vi "Process.vi"(8 "error in":errorcluster, 11 "ZMQ":refnum<class "ZMQ_SMO.lvclass">) -> (0 "error out":errorcluster, 3 "ZMQ out":refnum<class "ZMQ_SMO.lvclass">)   [LabVIEW 2016, in "ZMQ_SMO.lvclass"]
doc: "---------------------------------------------------------------\nJKI State Machine Objects™\nhttp://jki.net/state-machine-objects/\nCopyright (C) 2005-2015, JKI <info@jki.net>\nALL RIGHTS RESERVED"
uses:
  ZMQ_SMO.lvclass
  C:/Program Files (x86)/National Instruments/LabVIEW 2016/vi.lib/JKI/JKI SMO/SMO/SMO.lvclass
  <vilib>/JKI/JKI SMO/SMO/Typedefs/Parent Call--Enum.ctl
  <vilib>/addons/zeromq/socket_type.ctl
  <vilib>/addons/zeromq/zmq_context.lvclass
  <vilib>/addons/zeromq/zmq_socket.lvclass
  ZMQ_SMO.lvclass/ZMQ_SMO.ctl
  <vilib>/addons/zeromq/socket_options.ctl
  <vilib>/addons/zeromq/poll_type.ctl
  <vilib>/addons/zeromq/zmq_poll_scalar.vi
  <vilib>/JKI/JKI SMO/SMO/SMO.lvclass
  <vilib>/addons/zeromq/zeromq.lvlib
panel:
  # "For instructions on how to use the JKI State Machine Objects, examples and video tutorials, visit:\nhttp://jki.net/state-machine-objects/\n\nJKI State Machine Objects™\nhttp://jki.net/state-machine-objects/\nCopyright (C) 2005-2015, JKI <info@jki.net>\nALL RIGHTS RESERVED"
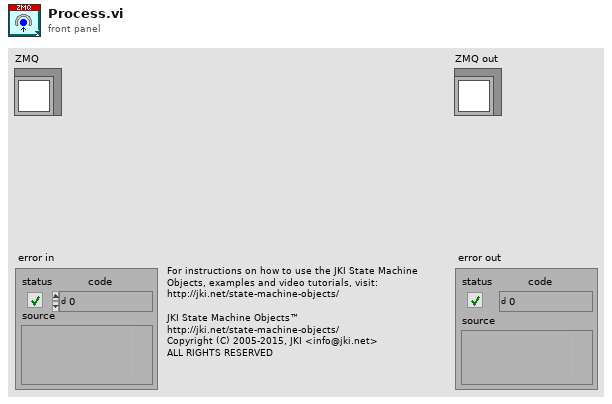
[diagram p1: front panel]
types:
  T1 = typedef "zeromq.lvlib/socket_type.ctl" = enum8{"ZMQ_PAIR", "ZMQ_PUB", "ZMQ_SUB", "ZMQ_REQ", "ZMQ_REP", "ZMQ_DEALER", "ZMQ_ROUTER", "ZMQ_PULL", "ZMQ_PUSH", "ZMQ_XPUB", "ZMQ_XSUB"}
  T2 = typedef "SMO.lvclass/Parent Call--Enum.ctl" = enum16{"Allows parent to run", "Does not request parent to run"}
  T3 = enum32{"invalid app kind", "Development System", "Run Time System", "Student Edition", "Embedded LabVIEW", "Evaluation", "Custom"}
  T4 = enum32{"Invalid", "Standard", "Closed", "Hidden", "Minimized", "Maximized"}
  T5 = enum32{"Bad", "Idle", "Run top level", "Running"}
  T6 = typedef "zeromq.lvlib/socket_options.ctl" = enum8{"NONE", "ZMQ_HWM", "<2>", "ZMQ_SWAP", "ZMQ_AFFINITY", "ZMQ_IDENTITY", "ZMQ_SUBSCRIBE", "ZMQ_UNSUBSCRIBE", "ZMQ_RATE", "ZMQ_RECOVERY_IVL", "ZMQ_MCAST_LOOP", "ZMQ_SNDBUF", "ZMQ_RCVBUF", "ZMQ_RCVMORE", "ZMQ_FD", "ZMQ_EVENTS", "ZMQ_TYPE", "ZMQ_LINGER", "ZMQ_RECONNECT_IVL", "ZMQ_BACKLOG", "ZMQ_RECOVERY_IVL_MSEC", "ZMQ_RECONNECT_IVL_MAX", "ZMQ_MAXMSGSIZE", "ZMQ_SNDHWM", "ZMQ_RCVHWM", "ZMQ_MULTICAST_HOPS", "<26>", "ZMQ_RCVTIMEO", "ZMQ_SNDTIMEO", "<29>", "<30>", "ZMQ_IPV4ONLY", "ZMQ_LAST_ENDPOINT", "ZMQ_ROUTER_MANDATORY", "ZMQ_TCP_KEEPALIVE", "ZMQ_TCP_KEEPALIVE_CNT", "ZMQ_TCP_KEEPALIVE_IDLE", "ZMQ_TCP_KEEPALIVE_INTVL", "ZMQ_TCP_ACCEPT_FILTER", "ZMQ_DELAY_ATTACH_ON_CONNECT", "ZMQ_XPUB_VERBOSE"}
  T7 = typedef "zeromq.lvlib/poll_type.ctl" = enum16{"None", "In", "Out", "In/Out"}
  T8 = typedef "ZMQ_SMO.lvclass/PrivateEvents--ZMQ.ZMQ_PublicMethod.ctl" = string[]
  T9 = typedef "ZMQ_ZMQ.lvclass/ZMQ Config.ctl" = cluster{"socket type":T1, "endpoint":string, "filter":string}
  T10 = cluster{"Core":cluster{"Current VI Reference":refnum<vi>, "Close Panel on Exit?":bool, "error":errorcluster}, "Self Reference":refnum<class "ZMQ_SMO.lvclass">, "parts":string[], "ZMQ context":refnum<class "zmq_context.lvclass">, "ZMQ socket":refnum<class "zmq_socket.lvclass">, "Config":T9, "to":i32}
  T11 = cluster{"Current VI Reference":refnum<vi>, "Close Panel on Exit?":bool, "error":errorcluster}
  T12 = typedef "SMO.lvclass/Protected Events.ctl" = cluster{"StopProcesses":refnum<user-event>, "AbortProcesses":refnum<user-event>, "Config Changed":refnum<user-event>, "Dependency":refnum<user-event>}
  T13 = typedef "ZMQ_SMO.lvclass/PrivateEvents--Cluster.ctl" = cluster{"ZMQ_message":refnum<user-event>}
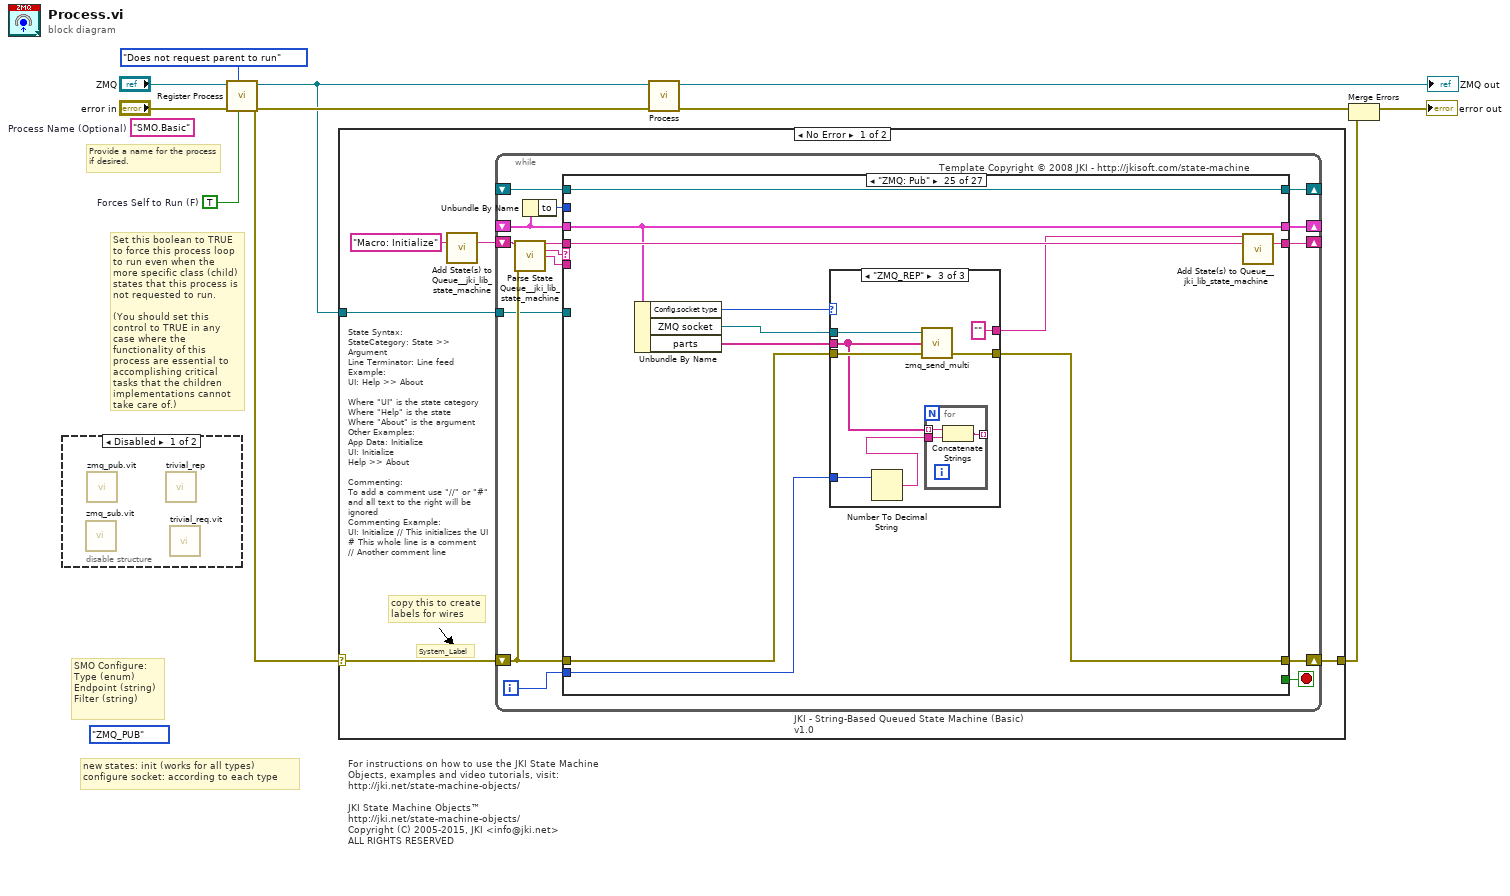
[diagram p0: block diagram]
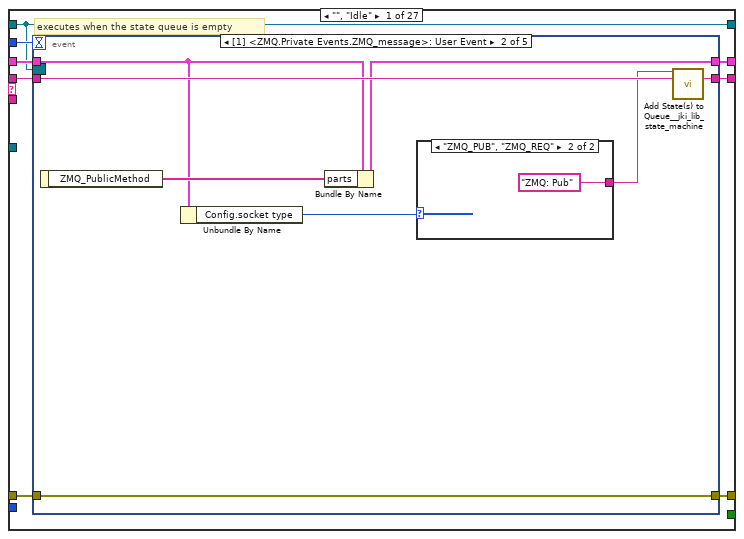
[diagram p3: hidden frame]
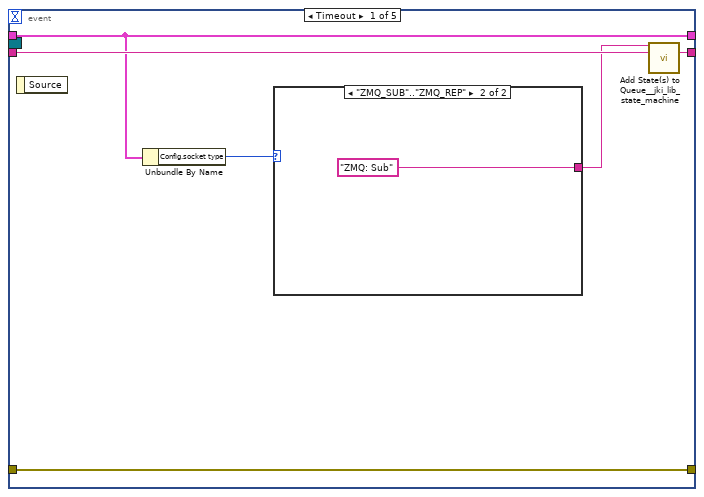
[diagram p4: hidden frame]
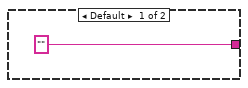
[diagram p5: hidden frame]
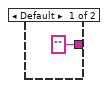
[diagram p6: hidden frame]
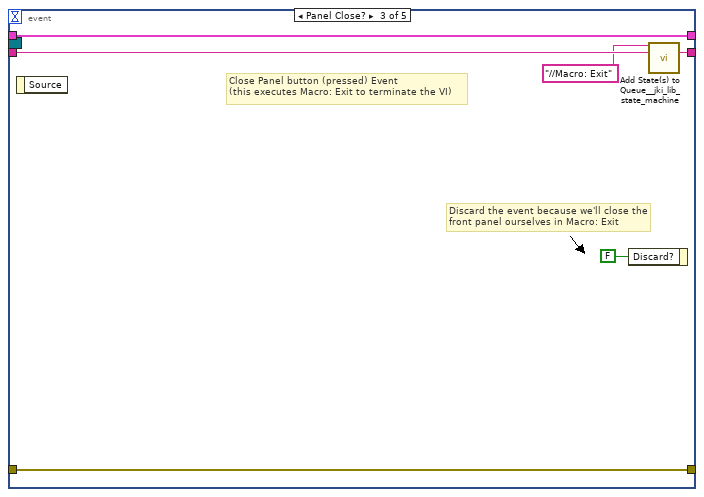
[diagram p7: hidden frame]
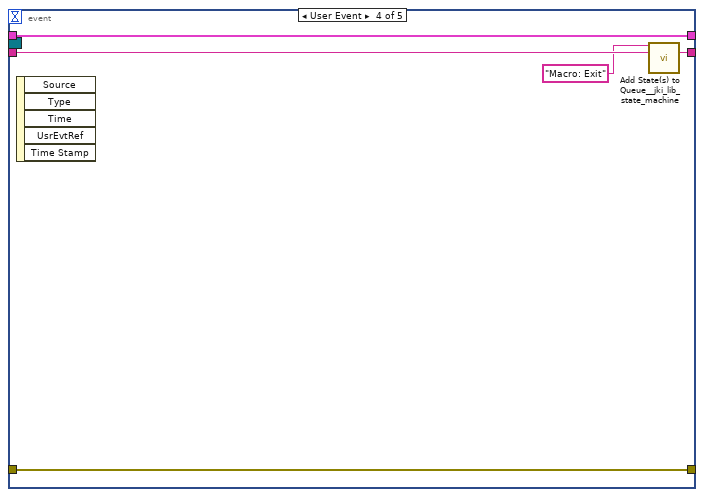
[diagram p8: hidden frame]
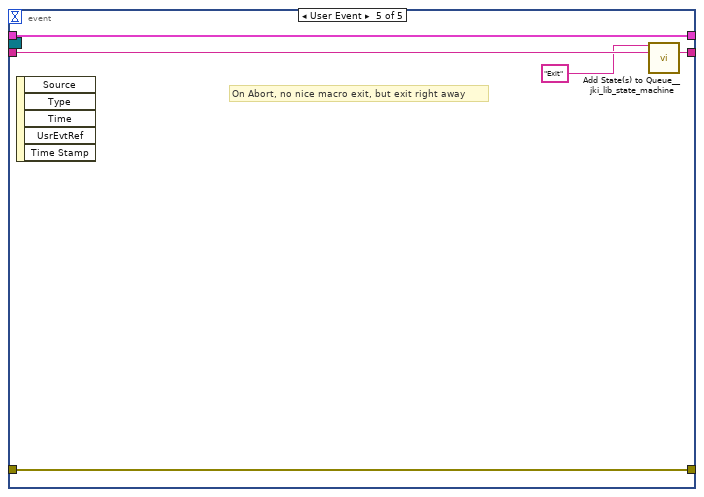
[diagram p9: hidden frame]
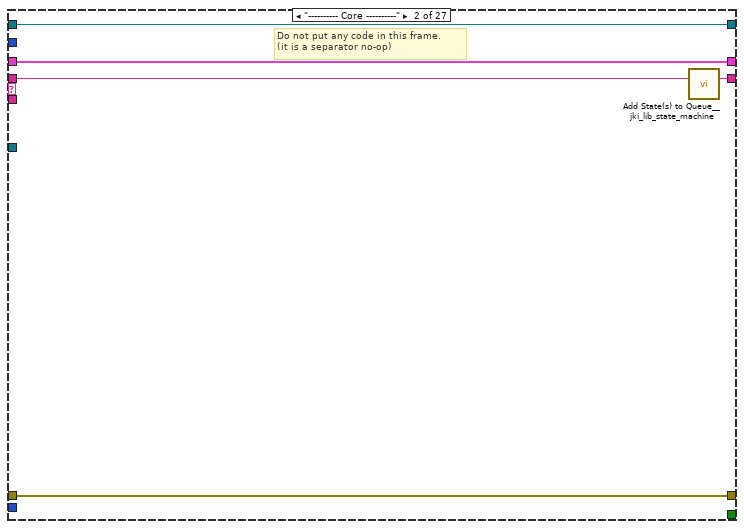
[diagram p10: hidden frame]
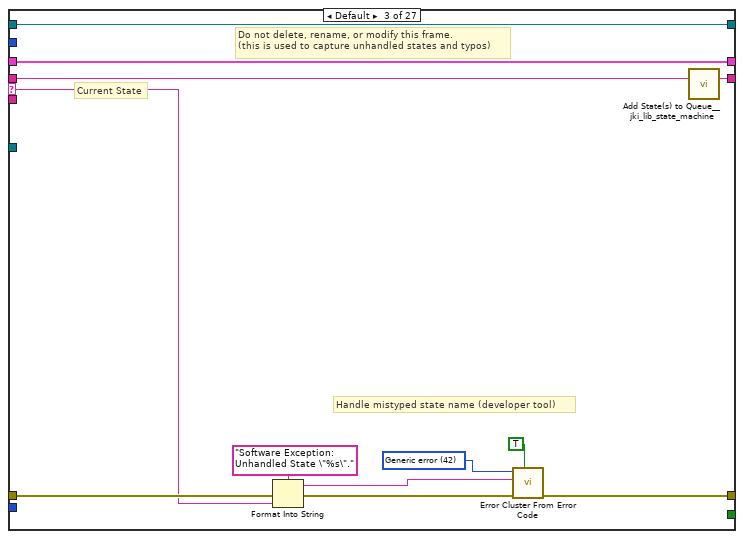
[diagram p11: hidden frame]
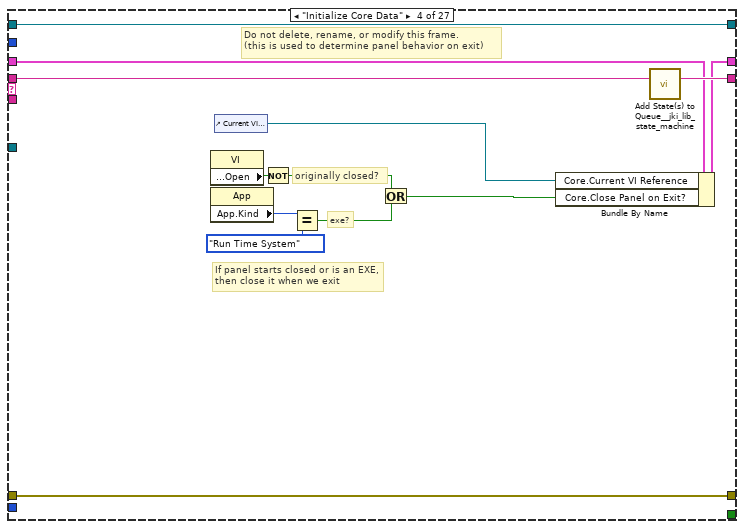
[diagram p12: hidden frame]
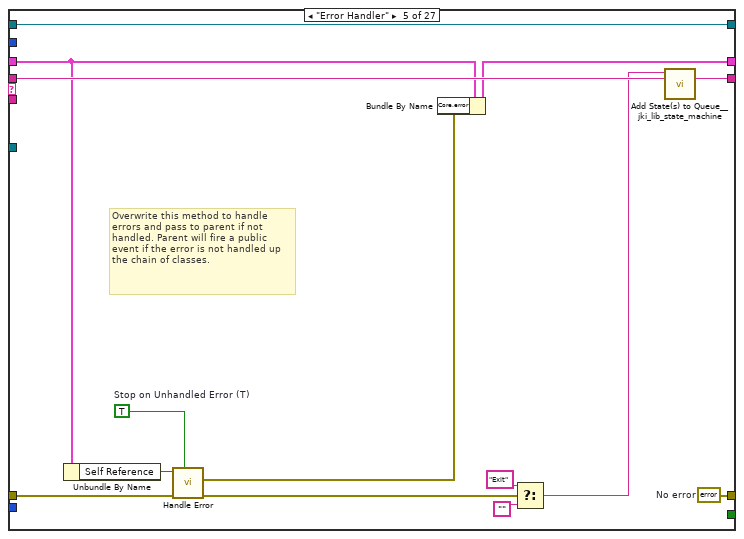
[diagram p13: hidden frame]
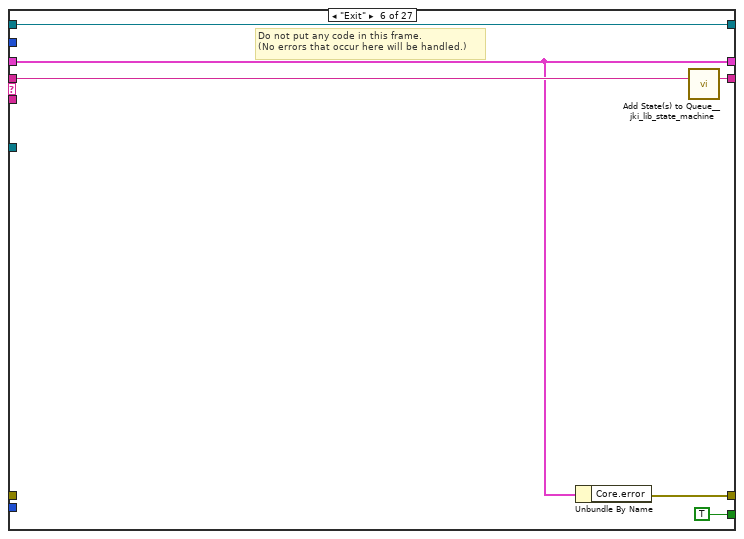
[diagram p14: hidden frame]
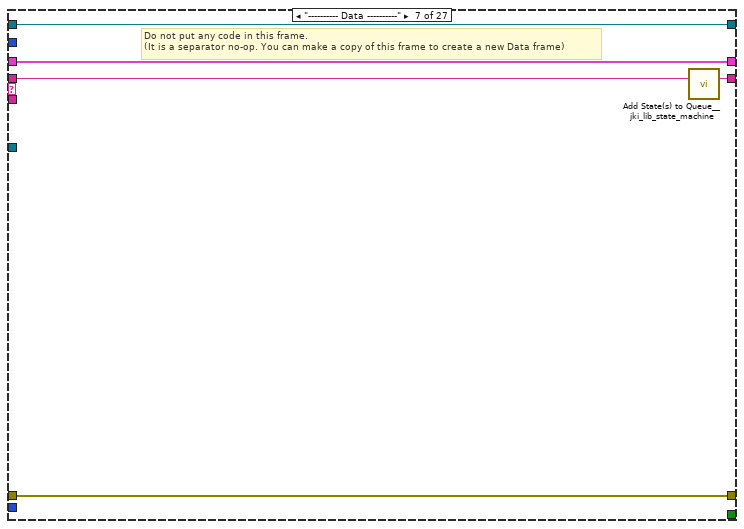
[diagram p15: hidden frame]
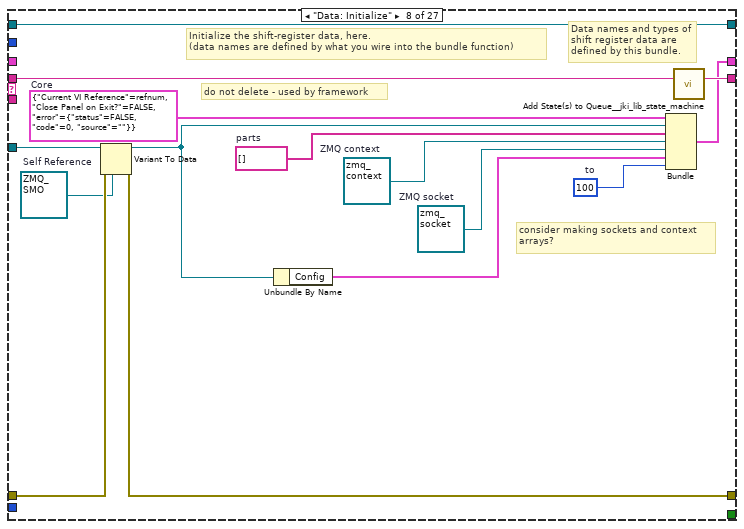
[diagram p16: hidden frame]
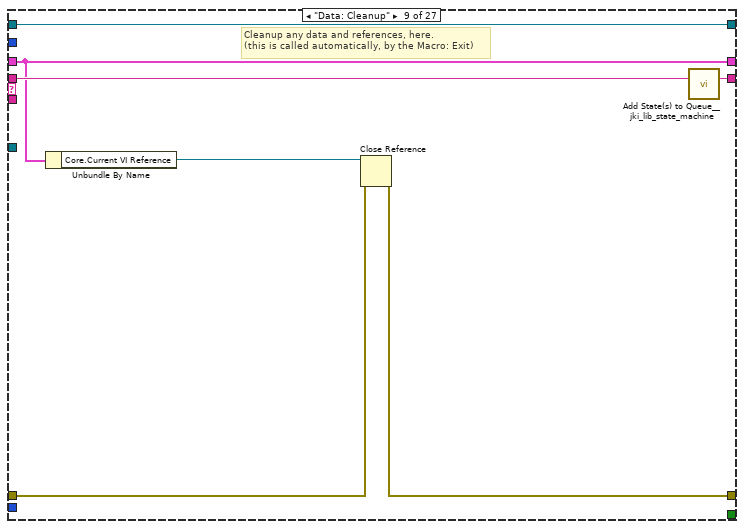
[diagram p17: hidden frame]
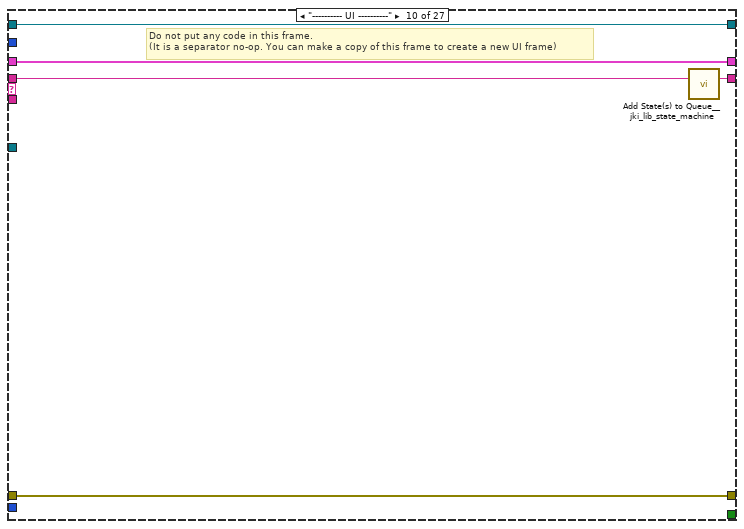
[diagram p18: hidden frame]
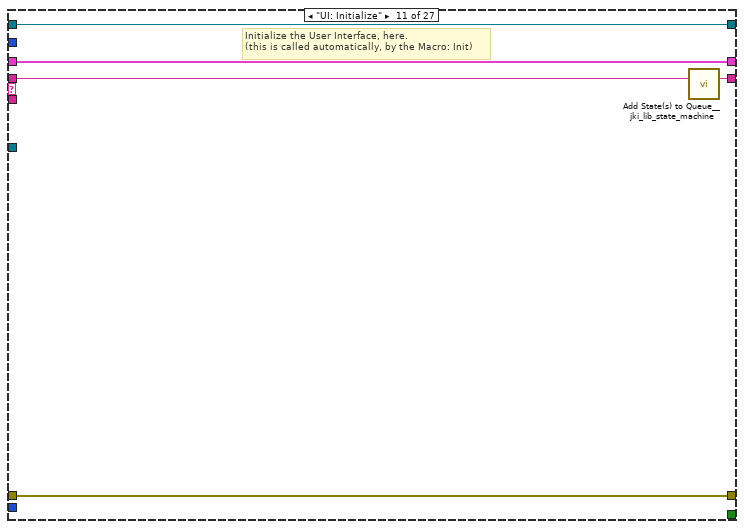
[diagram p19: hidden frame]
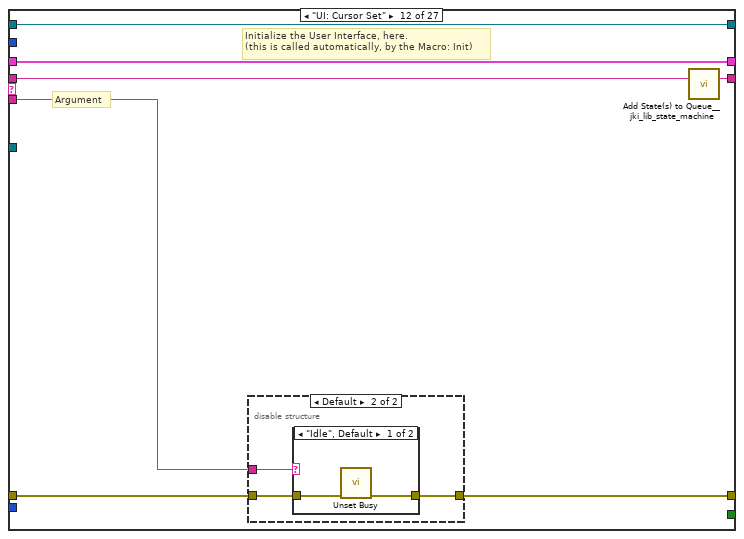
[diagram p20: hidden frame]
diagram:
  (unwired) socket_type."ZMQ_PUB" ("socket type")
  w1 = TRUE  # Forces Self to Run (F)
  (unwired) "SMO.Basic"  # Process Name (Optional)
  # "new states: init (works for all types)\nconfigure socket: according to each type"
  # "SMO Configure:\nType (enum)\nEndpoint (string)\nFilter (string)"
  # "Provide a name for the process\nif desired."
  # "Set this boolean to TRUE to force this process loop to run even when the more specific class (child) states that this process is not requested to run.\n\n(You should set this control to TRUE in any case where the functionality of this process are essential to accomplishing critical tasks that the children implementations cannot take care of.)"
  # "For instructions on how to use the JKI State Machine Objects, examples and video tutorials, visit:\nhttp://jki.net/state-machine-objects/\n\nJKI State Machine Objects™\nhttp://jki.net/state-machine-objects/\nCopyright (C) 2005-2015, JKI <info@jki.net>\nALL RIGHTS RESERVED"
  n1 = disable-structure shown="Disabled" {
    frame Disabled {
      n2 = call "zmq_sub.vit"() -> ()  [unwired: 12 in]
      n3 = call "zmq_pub.vit"() -> ()  [unwired: 12 in]
      n4 = call "trivial_rep.vi"() -> ()  [unwired: 12 in]
      n5 = call "trivial_req.vit"() -> ()  [unwired: 12 in]
    }
    frame Enabled {
    }
  }
  n6 = call <vilib>:"Register Process.vi"("Forces Self to Run (F)"=w1, "Parent Call"=Parent_Call--Enum."Does not request parent to run", "error in (no error)"="error in", "SMO"="ZMQ") -> ("error out"=w7:errorcluster, "SMO out"=w6:refnum<class "ZMQ_SMO.lvclass">)  [unwired: 6 in]
  n7 = case shown="No Error" w7 {
    selector: w7 -> [w12 w411]
    tunnel: w6 -> [w13 _]
    tunnel: [w11 w411] -> w3
    frame No Error {
      # "State Syntax:\nStateCategory: State >> Argument\nLine Terminator: Line feed\nExample:\nUI: Help >> About\n\nWhere \"UI\" is the state category\nWhere \"Help\" is the state\nWhere \"About\" is the argument\nOther Examples:\nApp Data: Initialize\nUI: Initialize\nHelp >> About\n\nCommenting:\nTo add a comment use \"//\" or \"#\" and all text to the right will be ignored\nCommenting Example:\nUI: Initialize // This initializes the UI\n# This whole line is a comment\n// Another comment line"
      # "copy this to create labels for wires"
      # "System_Label"
      n8 = call <vilib>:"Add State(s) to Queue__jki_lib_state_machine.vi"("State(s) in (\"\")"="Macro: Initialize") -> ("States Out"=w15:string)  [unwired: 14 in]
      n9 = while "JKI - String-Based Queued State Machine (Basic) v1.0" {
        shift-right: [w23] -> _
        shift-left: _ -> [w17]
        shift-right: [w26] -> w11
        shift-left: w12 -> [w22]
        shift-right: [w25] -> _
        shift-left: w15 -> [w27]
        tunnel: w13 -> [w21]
        shift-right: [w20] -> _
        shift-left: _ -> [w19]
        i -> [w16]
        stop <- w24 stop-if-true
        # "Template Copyright © 2008 JKI - http://jkisoft.com/state-machine"
        n10 = call <vilib>:"Parse State Queue__jki_lib_state_machine.vi"("State Queue"=w27, "Error In (no error)"=w22) -> ("Remaining States"=w29:string, "Current State"=w30:string, "Arguments"=w28:string)  [unwired: 11 in]
        n11 = Unbundle By Name(w17) -> ("to"=w18:i32)
        n12 = case shown="\"ZMQ: Pub\"" w30 {
          selector: w30 -> [_ _ w79 _ _ _ _ _ _ _ _ _ _ _ _ _ _ _ _ _ _ _ _ _ _ _ _]
          tunnel: w29 -> [w38 w77 w83 w102 w116 w122 w127 w142 w149 w154 w159 w166 w182 w214 w228 w242 w247 w258 w263 w276 w282 w287 w299 w312 w351 w381 w410]
          tunnel: w28 -> [_ _ _ _ _ _ _ _ _ _ _ w160 w176 _ _ _ _ _ _ _ _ _ _ _ _ _ _]
          tunnel: w17 -> [w36 w74 w81 w93 w110 w118 w124 _ w144 w151 w157 w164 w178 w211 w216 w233 w244 w255 w260 w274 w280 w285 w288 w308 w344 w378 w402]
          tunnel: [w35 w75 w85 w99 w111 w117 w125 w139 w145 w152 w156 w161 w179 w212 w226 w240 w245 w249 w261 w269 w278 w283 w292 w305 w345 w377 w405] -> w26
          tunnel: w22 -> [w34 w75 w84 w99 w112 _ w125 w140 w146 w152 w156 w162 w180 w212 w226 w240 w245 w250 w261 w270 w278 w283 w290 w306 w346 w371 w406]
          tunnel: [w37 w76 w82 w101 w115 w121 w126 w141 w148 w153 w158 w165 w181 w213 w227 w241 w246 w257 w262 w275 w281 w286 w298 w311 w350 w380 w409] -> w25
          tunnel: [_ _ _ _ _ TRUE _ _ _ _ _ _ _ _ _ _ _ _ _ _ _ _ _ _ _ _ _] -> w24
          tunnel: [w33 w74 w81 w100 w109 w118 w124 w128 w144 w151 w157 w164 w178 w211 w216 w233 w244 w255 w260 w274 w280 w285 w296 w309 w344 w378 w402] -> w23
          tunnel: w18 -> [w32 _ _ _ _ _ _ _ _ _ _ _ _ _ _ _ _ _ _ _ _ _ _ _ _ _ _]
          tunnel: w21 -> [_ _ _ _ _ _ _ w137 _ _ _ _ _ _ _ _ _ _ _ _ _ _ _ _ _ _ _]
          tunnel: [w31 w73 w78 w90 w114 w119 w123 w136 w143 w150 w155 w163 w175 w210 w225 w234 w243 w256 w259 w273 w279 w284 w297 w310 w349 w379 w408] -> w20
          tunnel: w19 -> [w31 w73 w78 w90 w114 w119 w123 w136 w143 w150 w155 w163 w175 w210 w225 w234 w243 w256 w259 _ w279 w284 w297 w310 w349 w379 w408]
          tunnel: w16 -> [_ _ _ _ _ _ _ _ _ _ _ _ _ _ _ _ _ _ _ _ _ _ _ _ w341 _ _]
          frame "", "Idle" {
            # "executes when the state queue is empty"
            n13 = event shown="[1] <ZMQ.Private Events.ZMQ_message>: User Event" {
              selector: w31 -> [_ _ _ _ _]
              dyn-events: _ -> [_ _ _ _ _]
              timeout: w32 -> [_ _ _ _ _]
              tunnel: w38 -> [w44 w54 w62 w67 w72]
              tunnel: [w43 w53 w61 w66 w71] -> w37
              tunnel: w36 -> [w42 w48 w59 w64 w69]
              tunnel: [w40 w49 w60 w65 w70] -> w35
              tunnel: w34 -> [w40 w49 w60 w65 w70]
              tunnel: [w42 w52 w59 w64 w69] -> w33
              event Timeout {
                n14 = event-data() -> ()  [unwired: 1 in, 1 out]
                n15 = Unbundle By Name(w42) -> ("Config.socket type"=w41:T1)
                n16 = case shown="\"ZMQ_SUB\"..\"ZMQ_REP\"" w41 {
                  tunnel: ["" ("string") "ZMQ: Sub" ("string")] -> w39
                  frame Default {
                  }
                  frame "ZMQ_SUB".."ZMQ_REP" {
                  }
                }
                n17 = call <vilib>:"Add State(s) to Queue__jki_lib_state_machine.vi"("State(s) in Front (\"\")"=w39, "State(s) in (\"\")"=w44) -> ("States Out"=w43:string)  [unwired: 13 in]
              }
              event User Event {
                n18 = event-data() -> ("ZMQ_PublicMethod"=w51:T8)  [unwired: 1 in]
                n19 = Unbundle By Name(w48) -> ("Config.socket type"=w47:T1)
                n20 = Bundle By Name(cluster=w48, "parts"=w51) -> (w52:T10)
                n21 = case shown="\"ZMQ_PUB\", \"ZMQ_REQ\"" w47 {
                  tunnel: ["" ("string") "ZMQ: Pub" ("string")] -> w50
                  frame Default {
                  }
                  frame "ZMQ_PUB", "ZMQ_REQ" {
                  }
                }
                n22 = call <vilib>:"Add State(s) to Queue__jki_lib_state_machine.vi"("State(s) in Front (\"\")"=w50, "State(s) in (\"\")"=w54) -> ("States Out"=w53:string)  [unwired: 13 in]
              }
              event Panel Close? {
                # "Discard the event because we'll close the front panel ourselves in Macro: Exit"
                # "Close Panel button (pressed) Event\n(this executes Macro: Exit to terminate the VI)"
                n23 = event-data() -> ()  [unwired: 1 in, 1 out]
                n24 = event-data("Discard?"=FALSE) -> ()  [unwired: 1 in, 1 out]
                n25 = call <vilib>:"Add State(s) to Queue__jki_lib_state_machine.vi"("State(s) in Front (\"\")"="//Macro: Exit", "State(s) in (\"\")"=w62) -> ("States Out"=w61:string)  [unwired: 13 in]
              }
              event User Event {
                n26 = event-data() -> ()  [unwired: 1 in, 5 out]
                n27 = call <vilib>:"Add State(s) to Queue__jki_lib_state_machine.vi"("State(s) in Front (\"\")"="Macro: Exit", "State(s) in (\"\")"=w67) -> ("States Out"=w66:string)  [unwired: 13 in]
              }
              event User Event {
                # "On Abort, no nice macro exit, but exit right away"
                n28 = event-data() -> ()  [unwired: 1 in, 5 out]
                n29 = call <vilib>:"Add State(s) to Queue__jki_lib_state_machine.vi"("State(s) in Front (\"\")"="Exit", "State(s) in (\"\")"=w72) -> ("States Out"=w71:string)  [unwired: 13 in]
              }
            }
          }
          frame "---------- Core ----------" {
            # "Do not put any code in this frame.\n(it is a separator no-op)"
            n30 = call <vilib>:"Add State(s) to Queue__jki_lib_state_machine.vi"("State(s) in (\"\")"=w77) -> ("States Out"=w76:string)  [unwired: 14 in]
          }
          frame Default {
            w88 = 42 items=["No error", "Argument error", "Memory is full", "Out of zone", "End of file", "File already open", "Generic file I/O error", "File not found", "File permission error", "Disk is full", "Duplicate path", "Too many files open", "System feature not enabled", "Resource file not found", "Cannot add resource", "Resource not found", "Image not found", "Image memory error", "Pen does not exist", "Config type invalid", "Config token not found", "Config parse error", "Config memory error", "Bad external code format", "Bad external code offset", "External code not present", "Null window", "Destroy window error", "Null menu", "Print aborted", "Bad print record", "Print driver error", "Windows error during printing", "Memory error during printing", "Print dialog error", "Generic print error", "Invalid device refnum", "Device not found", "Device parameter error", "Device unit error", "Cannot open device", "Device call aborted", "Generic error", "Cancelled by user", "Object ID too low", "Object ID too high", "Object not in heap", "Unknown heap", "Unknown object (invalid DefProc)", "Unknown object (DefProc not in table)", "Message out of range", "Invalid (null) method", "Unknown message", "Manager call not supported", "Bad address", "Network operation in progress", "Network operation timed out", "Connection is busy", "Network attribute not supported", "Network error", "Address in use", "System out of memory", "Connection aborted", "Connection refused", "Not connected", "Already connected", "Connection closed", "Initialization error (interapplication manager)", "Bad occurrence", "Wait on unbound occurrence handler", "Occurrence queue overflow", "Datalog type conflict", "Unused", "Unrecognized type (interapplication manager)", "Memory corrupt", "Failed to make temporary DLL", "Old CIN version", "Drag socket not found", "Failed to load drop-object", "Failed to register OLE object", "Failed to release OLE object", "Format specifier type mismatch", "Unknown format specifier", "Too few format specifiers", "Too many format specifiers", "Scan failed", "Newer CIN version", "Error converting to variant", "Runtime menu error", "Password tampered", "Variant attribute not found", "Incompatible variant data type", "Event data is not available", "Event Store is not present", "Occurrence is not found", "Event Queue is not created", "Event info is not available", "Refnum passed is NULL", "Error retrieving Class GUID", "Error retrieving CoClass GUID", "Error retrieving TypeLib GUID.", "Bad built application magic bytes.", "Specific driver is different from the specific driver associated with the Logical Name.", "There is no session opened to the class driver.", "Max Error", "MAX - Error with config objects", "MAX - Error loading configuration", "MAX - Group not supported"]
            # "Current State"
            # "Do not delete, rename, or modify this frame.\n(this is used to capture unhandled states and typos)"
            # "Handle mistyped state name (developer tool)"
            n31 = Format Into String(format string="Software Exception: Unhandled State \"%s\"." ("message"), error in=w84, w79) -> (resulting string=w87:string, error out=w86:errorcluster)  [unwired: 1 in]
            n32 = call <vilib>:"Error Cluster From Error Code.vi"("show call chain? (False)"=TRUE, "error in (no error)"=w86, "error message (\"\")"=w87, "error code (0)"=w88) -> ("error out"=w85:errorcluster)  [unwired: 5 in]
            n33 = call <vilib>:"Add State(s) to Queue__jki_lib_state_machine.vi"("State(s) in (\"\")"=w83) -> ("States Out"=w82:string)  [unwired: 14 in]
          }
          frame "Initialize Core Data" {
            # "Do not delete, rename, or modify this frame.\n(this is used to determine panel behavior on exit)"
            # "originally closed?"
            # "exe?"
            # "If panel starts closed or is an EXE, then close it when we exit"
            n34 = property class="VI"() -> ("Front Panel.Open"=w98:bool)  [unwired: 2 in, 2 out]
            n35 = property class="App"() -> ("App.Kind"=w97:T3)  [unwired: 2 in, 2 out]
            n36 = control-ref of="Current VI Reference"() -> (w91:refnum<vi>)
            n37 = Not(x=w98) -> (.not. x?=w95:bool)
            n38 = Equal?(x=w97, y=T3."Run Time System" ("Application:Kind")) -> (x = y?=w94:bool)
            n39 = Or(x=w95, y=w94) -> (x .or. y?=w92:bool)
            n40 = Bundle By Name(cluster=w93, "Core.Current VI Reference"=w91, "Core.Close Panel on Exit?"=w92) -> (w100:T10)
            n41 = call <vilib>:"Add State(s) to Queue__jki_lib_state_machine.vi"("State(s) in (\"\")"=w102) -> ("States Out"=w101:string)  [unwired: 14 in]
          }
          frame "Error Handler" {
            w103 = TRUE  # Stop on Unhandled Error (T)
            w111 = errorcluster {"status"=FALSE, "code"=0, "source"=""}  # No error
            # "Overwrite this method to handle errors and pass to parent if not handled. Parent will fire a public event if the error is not handled up the chain of classes."
            n42 = Unbundle By Name(w110) -> ("Self Reference"=w113:refnum<class "ZMQ_SMO.lvclass">)
            n43 = call-dynamic "Handle Error.vi"("Stop on Unhandled Error (T)"=w103, "error in"=w112, "SMO"=w113) -> ("handling error"=w104:errorcluster, "Unhandled error"=w107:errorcluster)  [unwired: 6 in, 1 out]
            n44 = Bundle By Name(cluster=w110, "Core.error"=w107) -> (w109:T10)
            n45 = Select(t="Exit", s=w104, f="") -> (s? t:f=w108:string)
            n46 = call <vilib>:"Add State(s) to Queue__jki_lib_state_machine.vi"("State(s) in Front (\"\")"=w108, "State(s) in (\"\")"=w116) -> ("States Out"=w115:string)  [unwired: 13 in]
          }
          frame "Exit" {
            # "Do not put any code in this frame.\n(No errors that occur here will be handled.)"
            n47 = Unbundle By Name(w118) -> ("Core.error"=w117:errorcluster)
            n48 = call <vilib>:"Add State(s) to Queue__jki_lib_state_machine.vi"("State(s) in (\"\")"=w122) -> ("States Out"=w121:string)  [unwired: 14 in]
          }
          frame "---------- Data ----------" {
            # "Do not put any code in this frame.\n(It is a separator no-op. You can make a copy of this frame to create a new Data frame)"
            n49 = call <vilib>:"Add State(s) to Queue__jki_lib_state_machine.vi"("State(s) in (\"\")"=w127) -> ("States Out"=w126:string)  [unwired: 14 in]
          }
          frame "Data: Initialize" {
            w129 = 100  # to
            w130 = string[] []  # parts
            w133 = refnum<class "zmq_socket.lvclass"> refnum  # ZMQ socket
            w134 = refnum<class "zmq_context.lvclass"> refnum  # ZMQ context
            w135 = T11 {"Current VI Reference"=refnum, "Close Panel on Exit?"=FALSE, "error"={"status"=FALSE, "code"=0, "source"=""}}  # Core
            w138 = refnum<class "ZMQ_SMO.lvclass"> refnum  # Self Reference
            # "consider making sockets and context\narrays?"
            # "do not delete - used by framework"
            # "Data names and types of shift register data are defined by this bundle."
            # "Initialize the shift-register data, here.\n(data names are defined by what you wire into the bundle function)"
            n50 = Variant To Data(error in=w140, type=w138, Variant=w137) -> (data=w132:refnum<class "ZMQ_SMO.lvclass">, error out=w139:errorcluster)
            n51 = Unbundle By Name(w132) -> ("Config"=w131:T9)
            n52 = Bundle("Core"=w135, "Self Reference"=w132, "parts"=w130, "ZMQ context"=w134, "ZMQ socket"=w133, "Config"=w131, "to"=w129) -> (w128:T10)  [unwired: 1 in]
            n53 = call <vilib>:"Add State(s) to Queue__jki_lib_state_machine.vi"("State(s) in (\"\")"=w142) -> ("States Out"=w141:string)  [unwired: 14 in]
          }
          frame "Data: Cleanup" {
            # "Cleanup any data and references, here.\n(this is called automatically, by the Macro: Exit)"
            n54 = Unbundle By Name(w144) -> ("Core.Current VI Reference"=w147:refnum<vi>)
            n55 = Close Reference(reference=w147, error in (no error)=w146) -> (error out=w145:errorcluster)
            n56 = call <vilib>:"Add State(s) to Queue__jki_lib_state_machine.vi"("State(s) in (\"\")"=w149) -> ("States Out"=w148:string)  [unwired: 14 in]
          }
          frame "---------- UI ----------" {
            # "Do not put any code in this frame.\n(It is a separator no-op. You can make a copy of this frame to create a new UI frame)"
            n57 = call <vilib>:"Add State(s) to Queue__jki_lib_state_machine.vi"("State(s) in (\"\")"=w154) -> ("States Out"=w153:string)  [unwired: 14 in]
          }
          frame "UI: Initialize" {
            # "Initialize the User Interface, here.\n(this is called automatically, by the Macro: Init)"
            n58 = call <vilib>:"Add State(s) to Queue__jki_lib_state_machine.vi"("State(s) in (\"\")"=w159) -> ("States Out"=w158:string)  [unwired: 14 in]
          }
          frame "UI: Cursor Set" {
            # "Argument"
            # "Initialize the User Interface, here.\n(this is called automatically, by the Macro: Init)"
            n59 = disable-structure shown="Default" {
              disable-tunnel: w162 -> [w167 w170]
              disable-tunnel: [w167 w169] -> w161
              disable-tunnel: w160 -> [_ w168]
              frame condition #0 {
              }
              frame condition #1 (active) {
                n60 = case shown="\"Idle\", Default" w168 {
                  tunnel: w170 -> [w172 w174]
                  tunnel: [w171 w173] -> w169
                  frame "Idle", Default {
                    n61 = call <vilib>:"Unset Busy.vi"("error in (no error)"=w172) -> ("error out"=w171:errorcluster)  [unwired: 10 in]
                  }
                  frame "Busy" {
                    n62 = call <vilib>:"Set Busy.vi"("error in (no error)"=w174) -> ("error out"=w173:errorcluster)  [unwired: 9 in, 1 out]
                  }
                }
              }
            }
            n63 = call <vilib>:"Add State(s) to Queue__jki_lib_state_machine.vi"("State(s) in (\"\")"=w166) -> ("States Out"=w165:string)  [unwired: 14 in]
          }
          frame "UI: Front Panel State" {
            # "Argument"
            # "Set Front Panel Open or Closed\n(Usage: \"UI: Front Panel State >> Open|Close\")"
            n64 = Unbundle By Name(w178) -> ("Core.Current VI Reference"=w177:refnum<vi>)
            n65 = disable-structure shown="Default" {
              disable-tunnel: w180 -> [w186 w209]
              disable-tunnel: [w185 w209] -> w179
              disable-tunnel: w177 -> [w184 _]
              disable-tunnel: w176 -> [w183 _]
              frame condition #0 (active) {
                n66 = case shown="\"Close\"" w183 {
                  tunnel: w186 -> [w190 w203]
                  tunnel: [w192 w204] -> w185
                  tunnel: w184 -> [w191 w201]
                  frame "Open", Default {
                    n67 = property class="VI"(reference=w191, error in=w190) -> (reference out=w188:refnum<vi>, error out=w189:errorcluster, "FP.State"=w187:T4)
                    n68 = case shown="\"Closed\"" w187 {
                      tunnel: [w195 w198] -> w192
                      tunnel: w189 -> [w194 w198]
                      tunnel: w188 -> [w193 _]
                      frame "Closed" {
                        n69 = invoke class="VI" method="FP.Open"(reference=w193, error in=w194, "Activate"=TRUE, "State"=T4."Standard") -> (error out=w195:errorcluster)  [unwired: 1 in, 4 out]
                      }
                      frame Default {
                      }
                    }
                  }
                  frame "Close" {
                    n70 = property class="VI"(reference=w201, error in=w203) -> (reference out=w200:refnum<vi>, error out=w202:errorcluster, "FP.State"=w199:T4)
                    n71 = case shown="Default" w199 {
                      tunnel: [w205 w208] -> w204
                      tunnel: w202 -> [w205 w207]
                      tunnel: w200 -> [_ w206]
                      frame "Invalid", "Closed" {
                      }
                      frame Default {
                        n72 = invoke class="VI" method="FP.Close"(reference=w206, error in=w207) -> (error out=w208:errorcluster)  [unwired: 1 in, 2 out]
                      }
                    }
                  }
                }
              }
              frame condition #1 {
              }
            }
            n73 = call <vilib>:"Add State(s) to Queue__jki_lib_state_machine.vi"("State(s) in (\"\")"=w182) -> ("States Out"=w181:string)  [unwired: 14 in]
          }
          frame "---------- Macro ----------" {
            # "Do not put any code in this frame.\n(It is a separator no-op. You can make a copy of this frame to create a new Macro frame)"
            n74 = call <vilib>:"Add State(s) to Queue__jki_lib_state_machine.vi"("State(s) in (\"\")"=w214) -> ("States Out"=w213:string)  [unwired: 14 in]
          }
          frame "Macro: Initialize" {
            w221 = "UI: Initialize\nUI: Front Panel State >> Close\nZMQ: Init\nZMQ: Config"  # UI: Initialize UI: Front Panel State >> Close ZMQ: Init ZMQ: Config
            w217 = "Process: Sync"
            # "Initialization Macro\n(This is called once, when the VI starts)"
            n75 = control-ref of="This VI"() -> (w219:refnum<vi>)
            n76 = property class="VI"(reference=w219) -> ("Exec.State"=w218:T5)  [unwired: 1 in, 2 out]
            n77 = Equal?(x=w218, y=T5."Run top level") -> (x = y?=w223:bool)
            n78 = Select(t=w217, s=w223, f="") -> ()  [unwired: 1 out]
            n79 = call <vilib>:"Add State(s) to Queue__jki_lib_state_machine.vi"("State(s) in Front (\"\")"="Data: Initialize\nInitialize Core Data\nEvents: Register", "State(s) in (\"\")"=w217, "State(s) at Back (\"\")"=w221) -> ("States Out"=w220:string)  [unwired: 12 in]
            n80 = call <vilib>:"Add State(s) to Queue__jki_lib_state_machine.vi"("State(s) in Front (\"\")"=w220, "State(s) in (\"\")"=w228) -> ("States Out"=w227:string)  [unwired: 13 in]
          }
          frame "Macro: Exit" {
            # "Exit Macro\n(This is called once, when the VI exits)"
            n81 = Unbundle By Name(w233) -> ("Core.Close Panel on Exit?"=w239:bool)
            n82 = Select(t="UI: Front Panel State >> Close", s=w239, f="") -> (s? t:f=w236:string)
            n83 = call <vilib>:"Add State(s) to Queue__jki_lib_state_machine.vi"("State(s) in Front (\"\")"="ZMQ: Exit\nData: Cleanup\nEvents: Unregister", "State(s) in (\"\")"="Process: Sync", "State(s) at Back (\"\")"="Exit") -> ("States Out"=w230:string)  [unwired: 12 in]
            n84 = call <vilib>:"Add State(s) to Queue__jki_lib_state_machine.vi"("State(s) in (\"\")"=w236, "State(s) at Back (\"\")"=w230) -> ("States Out"=w235:string)  [unwired: 13 in]
            n85 = call <vilib>:"Add State(s) to Queue__jki_lib_state_machine.vi"("State(s) in Front (\"\")"=w235, "State(s) in (\"\")"=w242) -> ("States Out"=w241:string)  [unwired: 13 in]
          }
          frame "---------- Process ----------" {
            # "Template Separator\n(You can make a copy of, or modify, this frame)"
            n86 = call <vilib>:"Add State(s) to Queue__jki_lib_state_machine.vi"("State(s) in (\"\")"=w247) -> ("States Out"=w246:string)  [unwired: 14 in]
          }
          frame "Process: Sync" {
            n87 = Unbundle By Name(w255) -> ("Self Reference"=w251:refnum<class "ZMQ_SMO.lvclass">)
            n88 = call <vilib>:"WaitOnProcessSync.vi"("error in (no error)"=w250, "SMO"=w251) -> ("error out"=w249:errorcluster, "Don't run?"=w254:bool)  [unwired: 7 in, 1 out]
            n89 = Select(t="Data: Cleanup\nEvents: Unregister\nExit", s=w254, f="") -> (s? t:f=w248:string)
            n90 = call <vilib>:"Add State(s) to Queue__jki_lib_state_machine.vi"("State(s) in Front (\"\")"=w248, "State(s) in (\"\")"=w258) -> ("States Out"=w257:string)  [unwired: 13 in]
          }
          frame "---------- Events ----------" {
            # "Template Separator\n(You can make a copy of, or modify, this frame)"
            n91 = call <vilib>:"Add State(s) to Queue__jki_lib_state_machine.vi"("State(s) in (\"\")"=w263) -> ("States Out"=w262:string)  [unwired: 14 in]
          }
          frame "Events: Register" {
            # "Expand to add\nmore events"
            n92 = Unbundle By Name(w274) -> ("Self Reference"=w271:refnum<class "ZMQ_SMO.lvclass">)
            n93 = call <vilib>:"GetProtectedEvents.vi"("SMO"=w271) -> ("error out"=w264:errorcluster, "SMO Protected Events"=w272:T12, "SMO out"=w267:refnum<class "ZMQ_SMO.lvclass">)  [unwired: 8 in]
            n94 = call "ZMQ.GetPrivateEvents.vi"("ZMQ"=w267) -> ("error out"=w266:errorcluster, "ZMQ.Private Events"=w265:T13)  [unwired: 8 in, 1 out]
            n95 = register-events(w272, w265) -> (reference out=w273:refnum<event-registration>, error out=w268:errorcluster)  [unwired: 2 in]
            n96 = Merge Errors(w264, w270, w268, w266) -> (w269:errorcluster)
            n97 = call <vilib>:"Add State(s) to Queue__jki_lib_state_machine.vi"("State(s) in (\"\")"=w276) -> ("States Out"=w275:string)  [unwired: 14 in]
          }
          frame "Events: Unregister" {
            n98 = Unregister For Events(event registration refnum=w279, error in=w278) -> (error out=w277:errorcluster)
            n99 = call <vilib>:"Clear Errors.vi"("error in (no error)"=w277) -> ()  [unwired: 5 in, 2 out]
            n100 = call <vilib>:"Add State(s) to Queue__jki_lib_state_machine.vi"("State(s) in (\"\")"=w282) -> ("States Out"=w281:string)  [unwired: 14 in]
          }
          frame "---------- ZMQ ----------" {
            n101 = call <vilib>:"Add State(s) to Queue__jki_lib_state_machine.vi"("State(s) in (\"\")"=w287) -> ("States Out"=w286:string)  [unwired: 14 in]
          }
          frame "ZMQ: Init" {
            n102 = Unbundle By Name(w288) -> ("Config.socket type"=w289:T1)
            n103 = call <vilib>:"zmq_ctx_create.vi"("error in"=w290) -> ("error out"=w291:errorcluster, "context out"=w295:refnum<class "zmq_context.lvclass">)  [unwired: 3 in]
            n104 = call <vilib>:"zmq_socket.vi"("error in"=w291, "socket type"=w289, "context in"=w295) -> ("error out"=w292:errorcluster, "socket out"=w294:refnum<class "zmq_socket.lvclass">, "context out"=w293:refnum<class "zmq_context.lvclass">)  [unwired: 2 in]
            n105 = Bundle By Name(cluster=w288, "ZMQ context"=w293, "ZMQ socket"=w294) -> (w296:T10)
            n106 = call <vilib>:"Add State(s) to Queue__jki_lib_state_machine.vi"("State(s) in (\"\")"=w299) -> ("States Out"=w298:string)  [unwired: 14 in]
          }
          frame "ZMQ: Config" {
            # "add other modes: REP, REQ, etc"
            n107 = Unbundle By Name(w308) -> ("Config.socket type"=w303:T1, "ZMQ socket"=w307:refnum<class "zmq_socket.lvclass">, "Config.endpoint"=w302:string, "Config.filter"=w300:string)
            n108 = case shown="\"ZMQ_REQ\"" w303 {
              tunnel: w307 -> [w318 w325 w334 w340]
              tunnel: w306 -> [w317 w323 w332 w339]
              tunnel: w302 -> [w316 w324 w333 w338]
              tunnel: [w315 w322 w330 w337] -> w305
              tunnel: [w314 w320 w329 w336] -> w304
              tunnel: [-1 ("to") 100 ("to") 100 ("to") 1 ("to")] -> w301
              tunnel: w300 -> [_ w319 _ _]
              frame "ZMQ_PUB", Default {
                n109 = call <vilib>:"zmq_bind.vi"("error in"=w317, "endpoint"=w316, "socket in"=w318) -> ("error out"=w315:errorcluster, "socket out"=w314:refnum<class "zmq_socket.lvclass">)  [unwired: 1 in]
              }
              frame "ZMQ_SUB" {
                n110 = call <vilib>:"zmq_connect.vi"("error in"=w323, "endpoint"=w324, "socket in"=w325) -> ("error out"=w326:errorcluster, "socket out"=w327:refnum<class "zmq_socket.lvclass">)  [unwired: 1 in]
                n111 = call <vilib>:"zmq_setsocketopt.vi"("error in"=w326, "value"=w319, "option"=socket_options."ZMQ_SUBSCRIBE", "socket in"=w327) -> ("error out"=w322:errorcluster, "socket out"=w320:refnum<class "zmq_socket.lvclass">)  [unwired: 2 in]
              }
              frame "ZMQ_REQ" {
                n112 = call <vilib>:"zmq_connect.vi"("error in"=w332, "endpoint"=w333, "socket in"=w334) -> ("error out"=w330:errorcluster, "socket out"=w329:refnum<class "zmq_socket.lvclass">)  [unwired: 1 in]
              }
              frame "ZMQ_REP" {
                n113 = call <vilib>:"zmq_bind.vi"("error in"=w339, "endpoint"=w338, "socket in"=w340) -> ("error out"=w337:errorcluster, "socket out"=w336:refnum<class "zmq_socket.lvclass">)  [unwired: 1 in]
              }
            }
            n114 = Bundle By Name(cluster=w308, "to"=w301, "ZMQ socket"=w304) -> (w309:T10)
            n115 = call <vilib>:"Add State(s) to Queue__jki_lib_state_machine.vi"("State(s) in (\"\")"=w312) -> ("States Out"=w311:string)  [unwired: 14 in]
          }
          frame "ZMQ: Pub" {
            n116 = Unbundle By Name(w344) -> ("Config.socket type"=w343:T1, "ZMQ socket"=w347:refnum<class "zmq_socket.lvclass">, "parts"=w348:string[])
            n117 = case shown="\"ZMQ_REP\"" w343 {
              tunnel: w348 -> [_ w356 w357]
              tunnel: w347 -> [_ w355 w363]
              tunnel: w346 -> [w352 w354 w362]
              tunnel: [w352 w353 w360] -> w345
              tunnel: [_ _ "" ("State(s) in Front (\"\")")] -> w342
              tunnel: w341 -> [_ _ w359]
              frame Default {
              }
              frame "ZMQ_PUB", "ZMQ_REQ" {
                n118 = call <vilib>:"zmq_send_multi.vi"("error in"=w354, "parts"=w356, "socket in"=w355) -> ("error out"=w353:errorcluster)  [unwired: 1 in, 1 out]
              }
              frame "ZMQ_REP" {
                n119 = Number To Decimal String(number=w359) -> (decimal integer string=w358:string)  [unwired: 1 in]
                n120 = call <vilib>:"zmq_send_multi.vi"("error in"=w362, "parts"=w357, "socket in"=w363) -> ("error out"=w360:errorcluster)  [unwired: 1 in, 1 out]
                n121 = for {
                  tunnel: w357 -> [w366] mode=indexing
                  tunnel: w358 -> [w365]
                  tunnel: [w364] -> _ mode=indexing
                  n122 = Concatenate Strings(w366, w365) -> (w364:string)
                }
              }
            }
            n123 = call <vilib>:"Add State(s) to Queue__jki_lib_state_machine.vi"("State(s) in Front (\"\")"=w342, "State(s) in (\"\")"=w351) -> ("States Out"=w350:string)  [unwired: 13 in]
          }
          frame "ZMQ: Sub" {
            # "change polling to zmq_recv_event.vi"
            n124 = Unbundle By Name(w378) -> ("Config.socket type"=w369:T1, "Self Reference"=w373:refnum<class "ZMQ_SMO.lvclass">, "ZMQ socket"=w372:refnum<class "zmq_socket.lvclass">)
            n125 = Build Array(w372) -> (w370:refnum<class "zmq_socket.lvclass">[])
            n126 = call-poly <vilib>:"zmq_poll.vi"("error in"=w371, "poll type"=poll_type."In", "sockets"=w370) -> ("error out"=w376:errorcluster, "polled events"=w374:T7[])  [unwired: 1 in, 2 out]
            n127 = for {
              shift-right: [w389] -> _
              shift-left: w373 -> [w390]
              shift-right: [w387] -> w377
              shift-left: w376 -> [w388]
              tunnel: w370 -> [w386] mode=indexing
              tunnel: w374 -> [w385] mode=indexing
              tunnel: [w384] -> w368
              n128 = case shown="\"In\"" w385 {
                tunnel: w390 -> [w393 w399]
                tunnel: [w393 w398] -> w389
                tunnel: w388 -> [w392 w401]
                tunnel: [w392 w396] -> w387
                tunnel: w386 -> [_ w400]
                tunnel: ["" ("State(s) in Front (\"\")") "ZMQ: Pub" ("State(s) in Front (\"\")")] -> w384
                frame Default {
                }
                frame "In" {
                  n129 = call <vilib>:"zmq_recv_multi.vi"("error in"=w401, "socket in"=w400) -> ("error out"=w397:errorcluster, "parts"=w395:string[])  [unwired: 1 in, 1 out]
                  n130 = call "ZMQ.ZMQ_PublicEvent.vi"("error in (no error)"=w397, "ZMQ_PublicEvent"=w395, "ZMQ"=w399) -> ("error out"=w396:errorcluster, "ZMQ out"=w398:refnum<class "ZMQ_SMO.lvclass">)  [unwired: 7 in]
                }
              }
            }
            n131 = case shown="\"ZMQ_REP\"" w369 {
              tunnel: w368 -> [_ w383]
              tunnel: ["" ("State(s) in Front (\"\")") w383] -> w367
              frame Default {
              }
              frame "ZMQ_REP" {
              }
            }
            n132 = call <vilib>:"Add State(s) to Queue__jki_lib_state_machine.vi"("State(s) in Front (\"\")"=w367, "State(s) in (\"\")"=w381) -> ("States Out"=w380:string)  [unwired: 13 in]
          }
          frame "ZMQ: Exit" {
            n133 = Unbundle By Name(w402) -> ("ZMQ context"=w407:refnum<class "zmq_context.lvclass">, "ZMQ socket"=w404:refnum<class "zmq_socket.lvclass">)
            n134 = call <vilib>:"zmq_close.vi"("error in"=w406, "socket"=w404) -> ("error out"=w403:errorcluster)  [unwired: 3 in]
            n135 = call <vilib>:"zmq_ctx_destroy.vi"("error in"=w403, "context in"=w407) -> ("error out"=w405:errorcluster)  [unwired: 3 in]
            n136 = call <vilib>:"Add State(s) to Queue__jki_lib_state_machine.vi"("State(s) in (\"\")"=w410) -> ("States Out"=w409:string)  [unwired: 14 in]
          }
        }
      }
    }
    frame Error {
    }
  }
  n137 = call-parent "Process.vi"("error in"=w7, "SMO"=w6) -> ("error out"=w4:errorcluster, "SMO out"=→"ZMQ out":refnum<class "ZMQ_SMO.lvclass">)  [unwired: 8 in]
  n138 = Merge Errors(w4, w3) -> (→"error out":errorcluster)
